vi "Configure Channel.vi"(8 "error in (no error)":errorcluster, 11 "Scope Base CFG in":refnum<class "Scope Base CFG.lvclass">) -> (0 "error out":errorcluster, 3 "Scope Base CFG out":refnum<class "Scope Base CFG.lvclass">)   [LabVIEW 2023, in "HAL.lvlib" / "Scope Base CFG.lvclass"]
uses:
  Scope Base CFG.lvclass
  Scope Base CFG.lvclass/Scope Base CFG.ctl
panel:
  out "Attributes out":string
  in  "Attributes":string
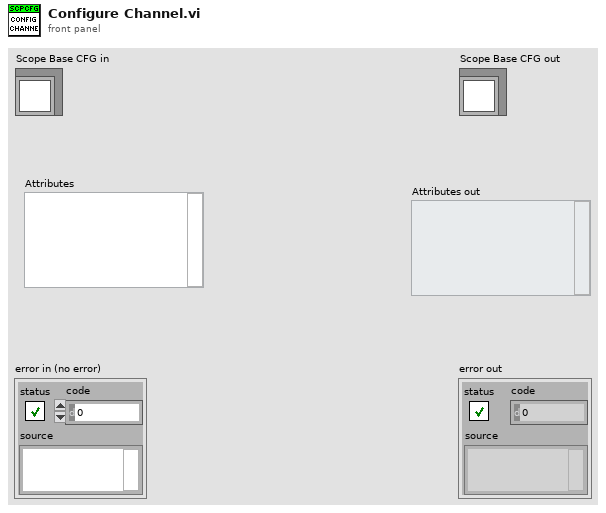
[diagram p1: front panel]
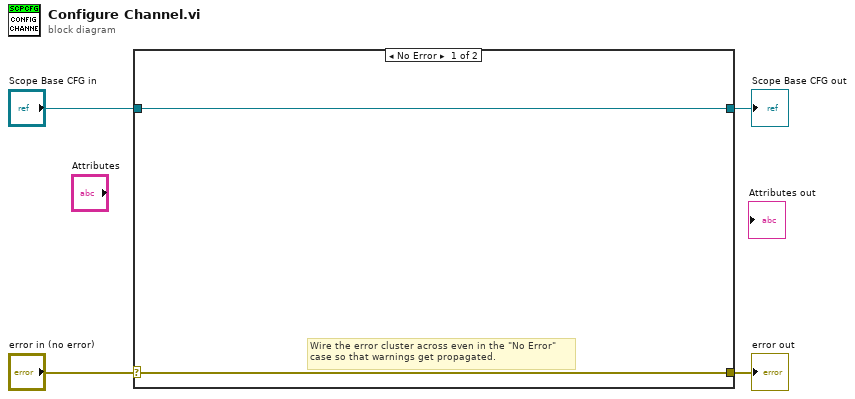
[diagram p0: block diagram]
diagram:
  n1 = case shown="No Error" "error in (no error)" {
    selector: "error in (no error)" -> [w5 w8]
    tunnel: [w5 w8] -> w3
    tunnel: [w6 w7] -> w1
    tunnel: "Scope Base CFG in" -> [w6 w7]
    frame No Error {
      # "Wire the error cluster across even in the \"No Error\"\ncase so that warnings get propagated."
    }
    frame Error {
    }
  }
  "error out" <- w3
  "Scope Base CFG out" <- w1
